vi "ellipse_theta_only_lm_objective.vi"(3 "output control":T1, 4 "data":variant, 5 "X":dbl[](array[numeric]), 6 "a":dbl[](array[numeric])) -> (0 "error out":errorcluster, 1 "f'(X,a)":dbl[][](array[numeric]), 2 "f(X,a)":dbl[](array[numeric]))   [LabVIEW 2017]
doc: "This template is the starting point for creating a model function to be passed to the Nonlinear Curve Fit.vi."
uses:
  <vilib>/gmath/NumericalOptimization/LM_output select.ctl
  typedefs/magnetic field fit.ctl
  <vilib>/gmath/NI_Gmath.lvlib
panel:
  # "a[0] = a, a[1] = b, a[2] = theta, a[3] = B0"
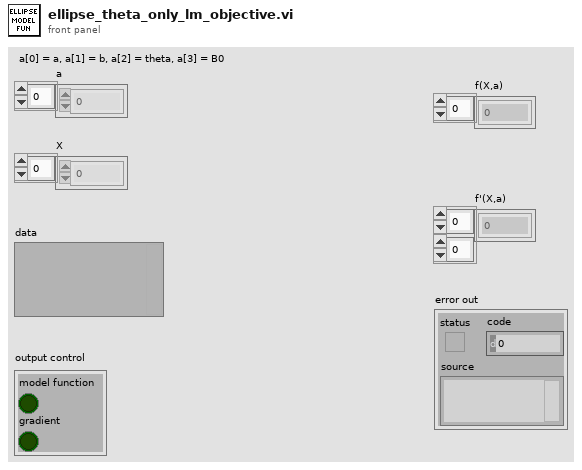
[diagram p1: front panel]
types:
  T1 = typedef "NI_Gmath.lvlib/LM_output select.ctl" = cluster{"model function":bool, "gradient":bool}
  T2 = typedef "magnetic field fit.ctl" = cluster{"a":dbl, "b":dbl, "theta":dbl, "scaling":dbl, "tilt_x":dbl, "tilt_y":dbl, "bx_offset":dbl, "by_offset":dbl, "bz_offset":dbl, "x_offset":dbl, "y_offset":dbl}
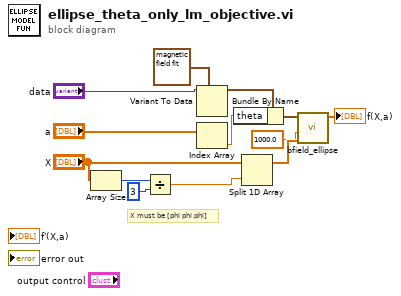
[diagram p0: block diagram]
diagram:
  # "X must be [phi phi phi]"
  n1 = Array Size(array="X") -> (size(s)=w12:i32)
  n2 = Divide(x=w12, y=3) -> (x/y=w10:dbl)
  n3 = Variant To Data(type=T2 {"a"=0.0, "b"=0.0, "theta"=0.0, "scaling"=0.0, "tilt_x"=0.0, "tilt_y"=0.0, "bx_offset"=0.0, "by_offset"=0.0, "bz_offset"=0.0, "x_offset"=0.0, "y_offset"=0.0} ("parameters"), Variant="data") -> (data=w4:T2)  [unwired: 1 in, 1 out]
  n4 = Index Array(array="a") -> (element=w2:dbl)  [unwired: 1 in]
  n5 = Bundle By Name(cluster=w4, "theta"=w2) -> (w1:T2)
  n6 = Split 1D Array(array="X", index=w10) -> (first subarray=w9:dbl[])  [unwired: 1 out]
  n7 = call "bfield_ellipse.vi"("phi"=w9, "L"=1000.0, "parameters"=w1) -> ("B(a,phi) as 1D"=→"f(X,a)":dbl[])  [unwired: 7 in, 1 out]
